vi "DashboardCore.vi"(10 "NT Viewer VIs":T1(array[cluster]), 11 "Plugin Info":T2) -> ()   [LabVIEW 2016]
uses:
  CorePluginInfo.ctl
  CoreDashGlobal.vi
panel:
  in  "TCP":refnum<k5>
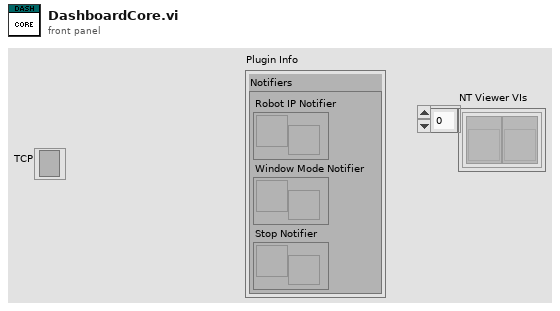
[diagram p1: front panel]
types:
  T1 = cluster{"VI Refnum":refnum<vi>, "TeleopSubPanel":refnum<vi>}[]
  T2 = typedef "CorePluginInfo.ctl" = cluster{"Notifiers":cluster{"Robot IP Notifier":refnum<notifier>, "Window Mode Notifier":refnum<notifier>, "Stop Notifier":refnum<notifier>}}
  T3 = cluster{"Error Strings":string, "Disable Counts":cluster{u16, u16}, "Rail Faults":cluster{u16, u16, u16}, "Robot IP":string, "DB Mode":u8, "Event Info":cluster{"Name":string, "Type":u8, "Number":u16, "Replay":u8}}
  T4 = cluster{"Storage":cluster{"Disk Free":u64, "RAM Block":u32, "RAM free":u32}, "CPU Utilization":cluster{"CPU % ISR":sgl, "CPU % Time Crit":sgl, "CPU % Timed Str":sgl, "CPU % High":sgl, "CPU % Above":sgl, "CPU % Normal":sgl, "CPU % Low":sgl}, "CAN":cluster{"% Bus Utilization":sgl, "Bus Off Cnt":u32, "TX_FIFO Full Cnt":u32, "Receive Error Cnt":u8, "Transmit Error Cnt":u8}, "HID":cluster{"HID Outputs":u32, "Rumble Low":u16, "Rumble High":u16}[]}
  T5 = cluster{"Status bits":cluster{"Test Mode":bool, "Autonomous":bool, "Enabled":bool, "Code Start":bool, "Brownout":bool, "Reserved 2":bool, "Reserved 3":bool, "E-Stop":bool}, "Code Trace":cluster{"Disabled":bool, "TeleOp":bool, "Auto":bool, "Test":bool}, "Controller Type":enum16{"unknown", "cRIO", "roboRio"}, "Code?":enum16{"unknown", "noCode", "code"}, "Battery V":dbl}
  T6 = cluster{"Control Bits":cluster{"TestMode":bool, "Autonomous":bool, "Enabled":bool, "FMS Present":bool, bool, bool, bool, "E-Stop":bool}, "Team Station ":u8, "Countdown":sgl, "Joystick Values":cluster{"Axes":dbl[], "Buttons":bool[], "POVs":i16[]}[]}
  T7 = enum8{"Tele-Op Disabled", "Tele-Op Enabled", "Auto Disabled", "Auto Enabled", "Test Disabled", "Test Enabled", "Disconnected", "No Code", "E-Stop"}
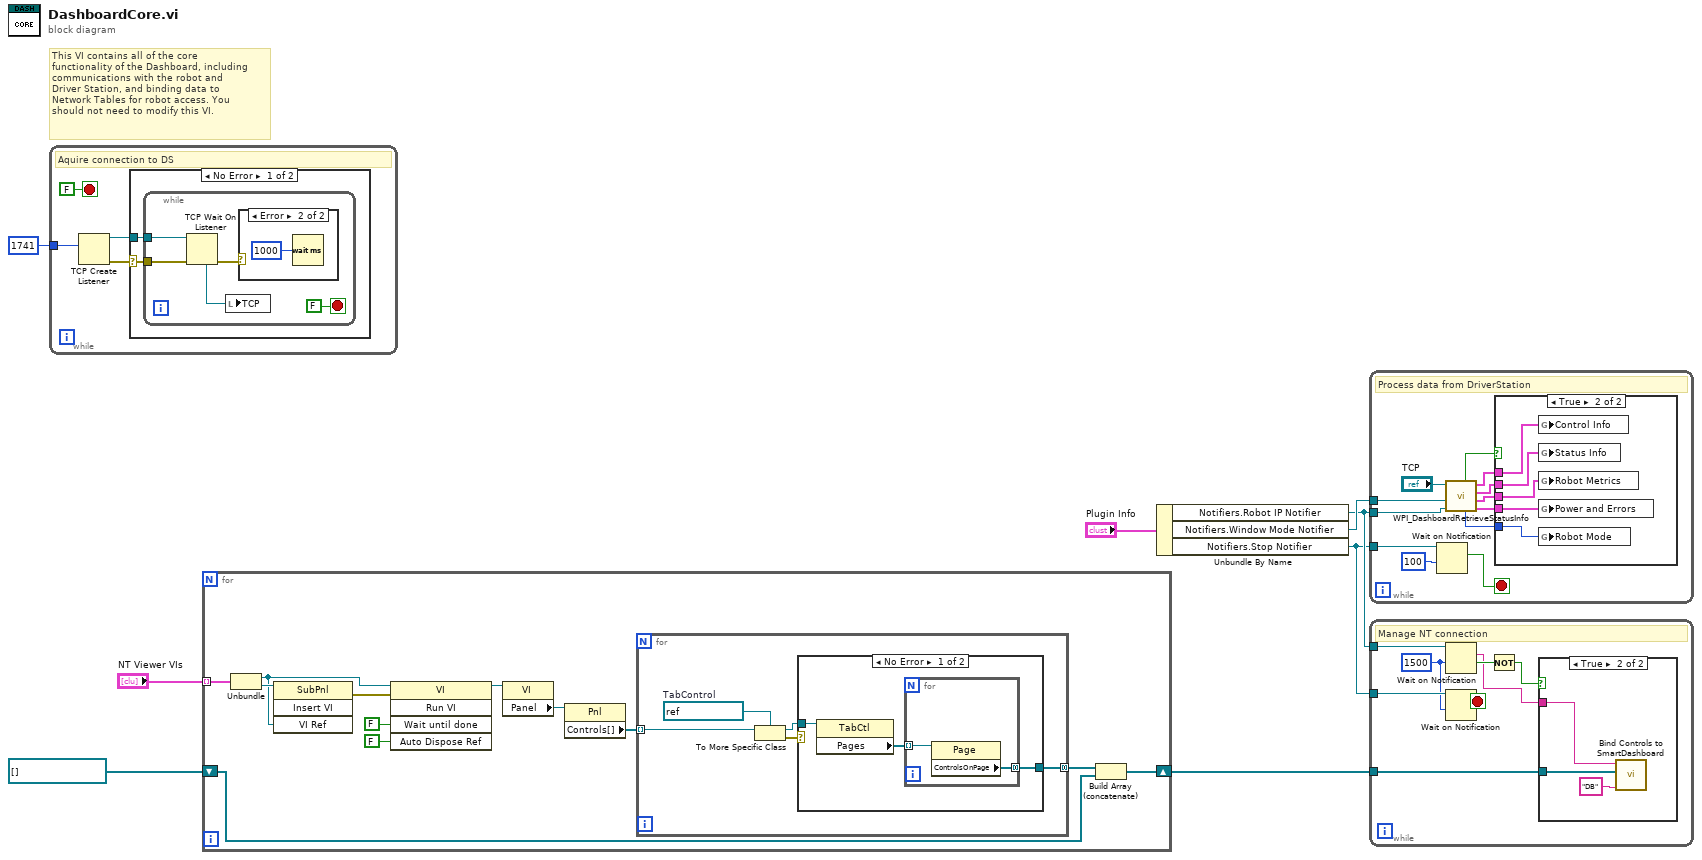
[diagram p0: block diagram]
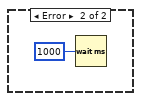
[diagram p5: hidden frame]
diagram:
  # "This VI contains all of the core\nfunctionality of the Dashboard, including\ncommunications with the robot and\nDriver Station, and binding data to \nNetwork Tables for robot access. You\nshould not need to modify this VI."
  n1 = while {
    tunnel: u16 1741 ("timeout ms (25000)") -> [w10]
    stop <- FALSE stop-if-true
    # "Aquire connection to DS"
    n2 = TCP Create Listener(10:w10) -> (0:w9:errorcluster, 3:w11:refnum<k5>)  [unwired: 4 in, 1 out]
    n3 = case shown="No Error" w9 {
      selector: w9 -> [w13 _]
      tunnel: w11 -> [w14 _]
      frame No Error {
        n4 = while {
          tunnel: w14 -> [w18]
          tunnel: w13 -> [w17]
          stop <- FALSE stop-if-true
          n5 = TCP Wait On Listener(8:w17, 11:w18) -> (0:w19:errorcluster, 4:w15:refnum<k5>)  [unwired: 2 in, 3 out]
          n6 = local write "TCP"(w15) -> ()
          n7 = case shown="Error" w19 {
            frame No Error {
            }
            frame Error {
              n8 = Wait (ms)(milliseconds to wait=u32 1000) -> ()  [unwired: 1 out]
            }
          }
        }
      }
      frame Error {
        n9 = Wait (ms)(milliseconds to wait=u32 1000) -> ()  [unwired: 1 out]
      }
    }
  }
  n10 = for {
    tunnel: "NT Viewer VIs" -> [w28] mode=indexing
    shift-right: [w29] -> w1
    shift-left: refnum<vi>[] [] ("Controls To Bind") -> [w30]
    n11 = Unbundle(w28) -> ("VI Refnum"=w23:refnum<vi>, "TeleopSubPanel"=w24:refnum<vi>)
    n12 = invoke class="SubPnl" method="Insert VI"(reference=w24, "VI Ref"=w23) -> (error out=w22:errorcluster)  [unwired: 2 in, 3 out]
    n13 = invoke class="VI" method="Run VI"(reference=w23, error in=w22, "Wait until done"=FALSE ("Wait Until Done"), "Auto Dispose Ref"=FALSE ("Auto Dispose Reference")) -> (reference out=w27:refnum<vi>)  [unwired: 1 in, 4 out]
    n14 = property class="VI"(reference=w27) -> ("Panel"=w33:refnum<vi>)  [unwired: 1 in, 2 out]
    n15 = property class="Pnl"(reference=w33) -> ("Controls[]"=w32:refnum<vi>[])  [unwired: 1 in, 2 out]
    n16 = for {
      tunnel: w32 -> [w38] mode=indexing
      tunnel: [w34] -> w31 mode=concatenating
      w37 = refnum<vi> refnum  # TabControl
      n17 = To More Specific Class(target class=w37, reference=w38) -> (specific class reference=w35:refnum<vi>, error out=w36:errorcluster)  [unwired: 1 in]
      n18 = case shown="No Error" w36 {
        tunnel: w35 -> [w41 _]
        tunnel: [w39 _] -> w34
        frame No Error {
          n19 = property class="TabCtl"(reference=w41) -> ("Pages"=w40:refnum<vi>[])  [unwired: 1 in, 2 out]
          n20 = for {
            tunnel: w40 -> [w43] mode=indexing
            tunnel: [w42] -> w39 mode=concatenating
            n21 = property class="Page"(reference=w43) -> ("ControlsOnPage"=w42:refnum<vi>[])  [unwired: 1 in, 2 out]
          }
        }
        frame Error {
        }
      }
    }
    n22 = Build Array (concatenate)(w31, w30) -> (w29:refnum<vi>[])
  }
  n23 = Unbundle By Name("Plugin Info") -> ("Notifiers.Robot IP Notifier"=w5:refnum<notifier>, "Notifiers.Window Mode Notifier"=w6:refnum<notifier>, "Notifiers.Stop Notifier"=w4:refnum<notifier>)
  n24 = while {
    tunnel: w6 -> [w54]
    tunnel: w5 -> [w53]
    tunnel: w4 -> [w45]
    stop <- w44 stop-if-true
    # "Process data from DriverStation"
    n25 = Wait on Notification(notifier=w45, timeout in ms (-1)=100) -> (notification=w44:bool)  [unwired: 2 in, 3 out]
    n26 = call <vilib>:"WPI_DashboardRetrieveStatusInfo.vi"("Binding Refnum"=w53, "Window Mode Notifier"=w54, "TCP Cnx"="TCP") -> ("Power and Errors"=w49:T3, "Robot Metrics"=w50:T4, "Status Info"=w51:T5, "Control Info"=w52:T6, "Robot Mode"=w48:T7, "Process?"=w47:bool)  [unwired: 3 in]
    n27 = case shown="True" w47 {
      tunnel: w52 -> [_ w60]
      tunnel: w51 -> [_ w59]
      tunnel: w50 -> [_ w58]
      tunnel: w49 -> [_ w57]
      tunnel: w48 -> [_ w56]
      frame False {
      }
      frame True {
        n28 = global write "CoreDashGlobal.vi" "Control Info"(w60) -> ()
        n29 = global write "CoreDashGlobal.vi" "Status Info"(w59) -> ()
        n30 = global write "CoreDashGlobal.vi" "Robot Metrics"(w58) -> ()
        n31 = global write "CoreDashGlobal.vi" "Power and Errors"(w57) -> ()
        n32 = global write "CoreDashGlobal.vi" "Robot Mode"(w56) -> ()
      }
    }
  }
  n33 = while {
    tunnel: w5 -> [w68]
    tunnel: w4 -> [w64]
    tunnel: w1 -> [w61]
    stop <- w62 stop-if-true
    w63 = 1500 ("timeout in ms (-1)")
    # "Manage NT connection"
    n34 = Wait on Notification(notifier=w68, timeout in ms (-1)=w63) -> (notification=w65:string, timed out?=w67:bool)  [unwired: 2 in, 2 out]
    n35 = Wait on Notification(notifier=w64, timeout in ms (-1)=w63) -> (notification=w62:bool)  [unwired: 2 in, 3 out]
    n36 = Not(x=w67) -> (.not. x?=w66:bool)
    n37 = case shown="True" w66 {
      tunnel: w65 -> [_ w69]
      tunnel: w61 -> [_ w70]
      frame False {
      }
      frame True {
        n38 = call <vilib>:"Bind Controls to SmartDashboard.vi"("Client Name"="DB", "Bound Control Refs"=w70, "Server IP Address"=w69) -> ()  [unwired: 9 in]
      }
    }
  }
